vi "VNA_Easy_Loop.vi"(4 "Power (dbm)":dbl=-19.0, 5 "Transport":refnum<class "Transport.lvclass">, 6 "stop/span":dbl=600000000.0 format="%.2p", 7 "VNA Address":refnum<visa-resource-name>="GPIB0::15::INSTR", 8 "start/center":dbl=400000000.0 format="%.2p", 9 "sweep type (0 : linear)":u16(ring) items=["linear sweep", "logarithmic sweep", "frequency list", "CW time sweep", "power sweep"], 10 "sweep time (sec)":dbl=1.0 format="%.2f", 11 "num points":u16(ring)=8 items=["3", "11", "21 ('20) / 26 ('53)", "51", "101", "201", "401", "801", "1601"]) -> (2 "Polar plot":cluster{dbl[], sgl[]}[](graph))   [LabVIEW 2019]
uses:
  <userlib>/LevyLab/Transport/Transport/Transport.lvclass/Transport.ctl
  <userlib>/LevyLab/Transport/Control Experiment/Control Experiment.lvclass/Control Experiment.ctl
  <userlib>/LevyLab/Instrument Framework/Instrument Types/Cryostat/Instrument.Cryostat.lvclass
  <instrlib>/Agilent 87XX Series/Agilent 87XX Series.lvlib
  <userlib>/LevyLab/Transport/Control Experiment/Control Experiment.lvclass
  <userlib>/LevyLab/Transport/Transport/Transport.lvclass
panel:
  out "Data 2":cluster{dbl[], dbl[]}[](graph)
  out "B Field (T)":dbl=0.0002
  out "Temperature (K)":dbl=0.05877533421575553
  in  "Vg (V)":dbl
  in  "Ids (mA)":dbl=9.5
  in  "Vds (V)":dbl=1.3
  in  "Experiment Description":string="Vbg (1Gohm)=AO6 = P_pump = -20dBm to -5dBm, 0.1 dBm\n wait time 2s\nF_pump=2f0 = 900Mhz\n\nVbg(AO6) = 0V\nB=0T\nP_vna = -19.0 dBm (resonance at 488MHz with no pump)\n400MHz to 600MHz\nVd: 1.3V\nId: 9.5mA"
  in  "Experiment Folder":string="22-Vbgpump2f_Psweep_highPvna"
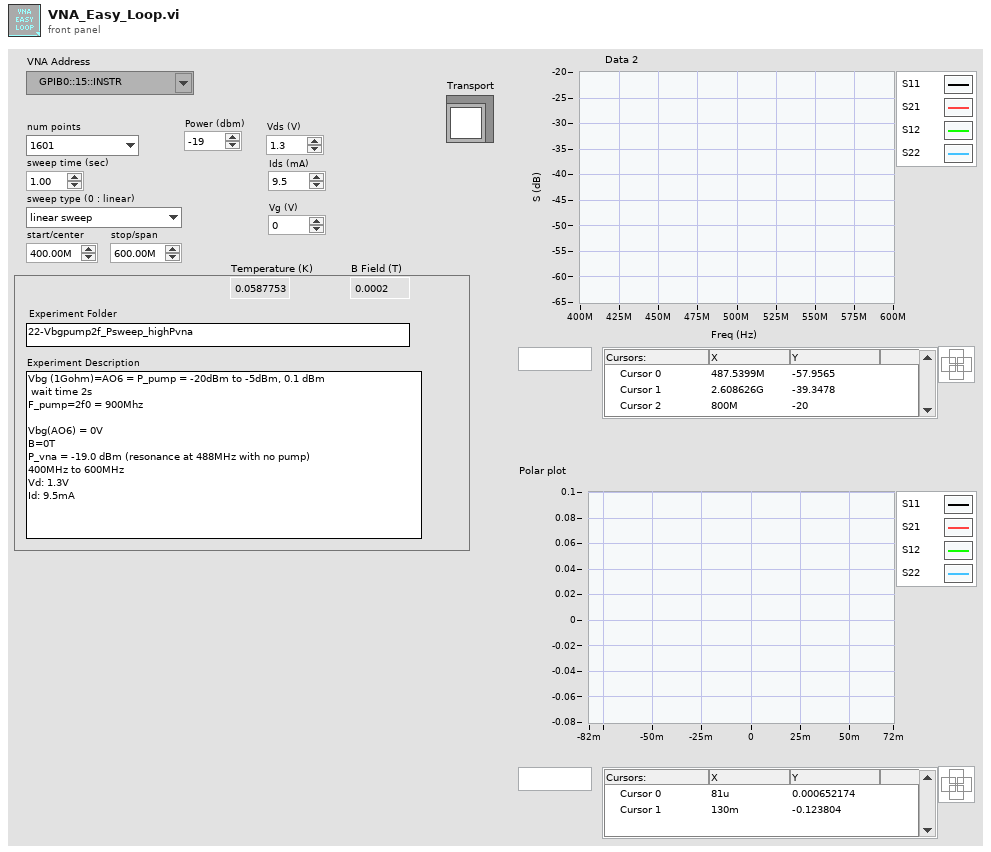
[diagram p1: front panel]
types:
  T1 = enum32{"Bad", "Idle", "Run top level", "Running"}
  T2 = typedef "Control Experiment.lvclass/Instruments--cluster.ctl" = cluster{"KH7008":refnum<class "Instrument.KH7008.lvclass">[], "Lockin":refnum<class "Instrument.Lockin.lvclass">, "Temperature":refnum<class "Instrument.Cryostat.lvclass">, "Magnet":refnum<class "Instrument.Cryostat.lvclass">, "Rotator":refnum<class "Instrument.Cryostat.lvclass">, "Level":refnum<class "Instrument.Cryostat.lvclass">, "Capacitance Bridge":refnum<class "Instrument.CBridge.lvclass">, "Delay Line":refnum<class "Instrument.DelayLine.lvclass">, "Strain Cell":refnum<class "Instrument.Strain.lvclass">, "VNA":refnum<class "Instrument.VNA.lvclass">, "Voltage Source":refnum<class "Instrument.VSource.lvclass">}
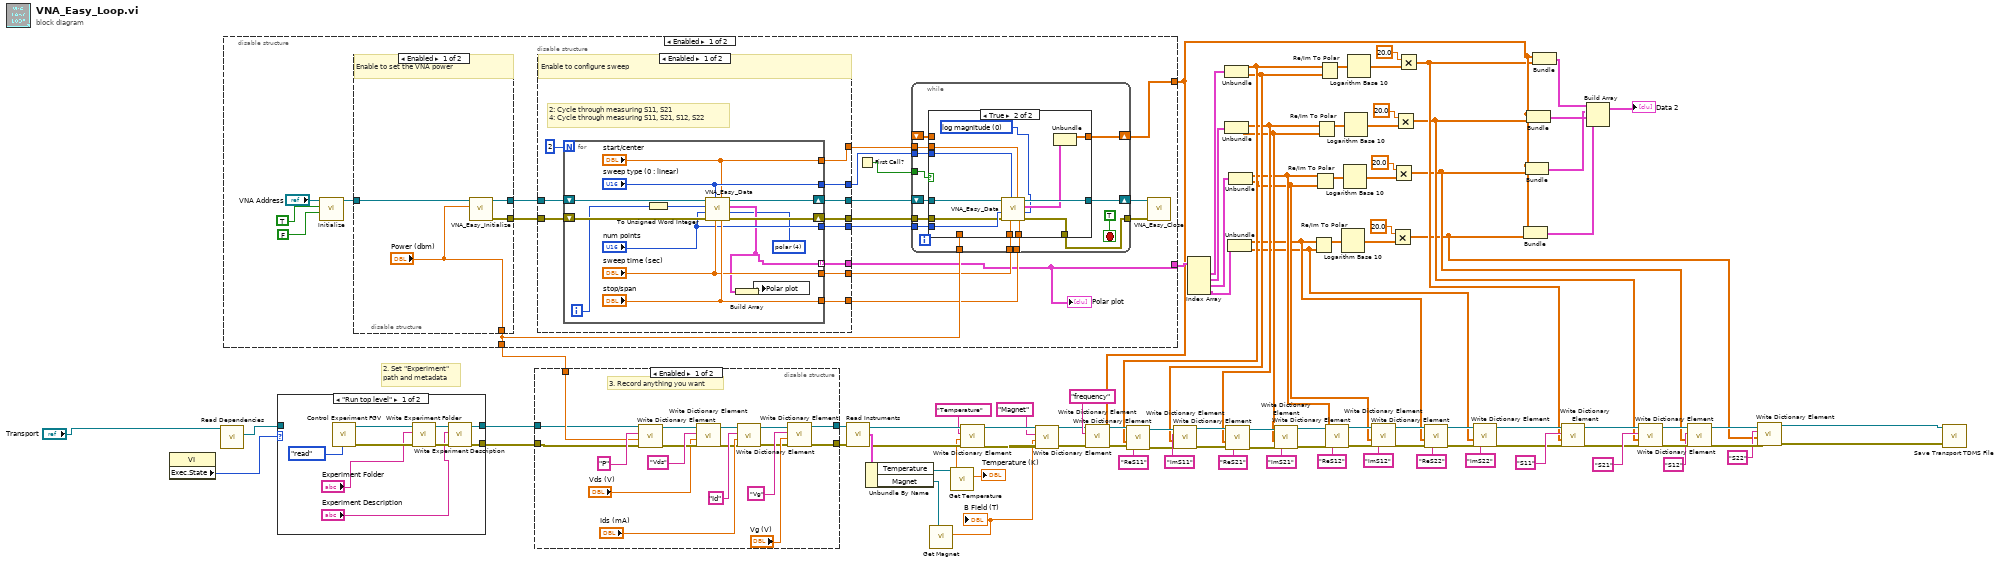
[diagram p0: block diagram]
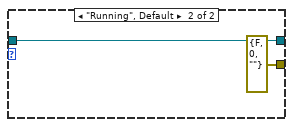
[diagram p2: hidden frame]
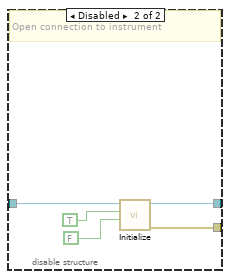
[diagram p5: hidden frame]
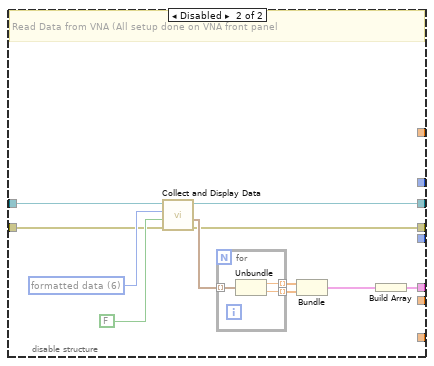
[diagram p6: hidden frame]
diagram:
  # "2. Set \"Experiment\"\npath and metadata"
  n1 = property class="VI"() -> ("Exec.State"=w62:T1)  [unwired: 2 in, 2 out]
  n2 = call <userlib>:"Read Dependencies.vi"("Transport"="Transport") -> ("C.E."=w58:refnum<class "Control Experiment.lvclass">)  [unwired: 8 in, 2 out]
  n3 = disable-structure shown="Enabled" {
    disable-tunnel: [w97 _] -> w57
    disable-tunnel: [w106 _] -> w88
    disable-tunnel: [w107 _] -> w15
    frame Enabled {
      n4 = call <instrlib>:"Initialize.vi"("reset"=FALSE, "ID query"=TRUE, "VISA resource name"="VNA Address") -> ("VISA resource name out"=w110:refnum<visa-resource-name>)  [unwired: 7 in, 1 out]
      n5 = disable-structure shown="Enabled" {
        disable-tunnel: w110 -> [w147 w150]
        disable-tunnel: [w146 w148] -> w114
        disable-tunnel: [w145 w149] -> w113
        disable-tunnel: ["Power (dbm)" _] -> w106
        frame Enabled {
          # "Enable to set the VNA power"
          n6 = call "VNA_Easy_Initialize.vi"("Power (dbm)"="Power (dbm)", "VISA Refnum in"=w147) -> ("error out"=w145:errorcluster, "VISA Refnum out"=w146:refnum<visa-resource-name>)  [unwired: 8 in]
        }
        frame Disabled {
          # "Open connection to instrument"
          n7 = call <instrlib>:"Initialize.vi"("reset"=FALSE, "ID query"=TRUE, "VISA resource name"=w150) -> ("error out"=w149:errorcluster, "VISA resource name out"=w148:refnum<visa-resource-name>)  [unwired: 7 in]
        }
      }
      n8 = disable-structure shown="Enabled" {
        disable-tunnel: w114 -> [w163 w182]
        disable-tunnel: w113 -> [w162 w183]
        disable-tunnel: [w161 w180] -> w105
        disable-tunnel: [w160 w181] -> w109
        disable-tunnel: [w159 w178] -> w97
        disable-tunnel: [w157 _] -> w103
        disable-tunnel: [w156 _] -> w102
        disable-tunnel: [w155 _] -> w101
        disable-tunnel: [w154 _] -> w100
        disable-tunnel: [w153 _] -> w99
        frame Enabled {
          # "2: Cycle through measuring S11, S21\n4: Cycle through measuring S11, S21, S12, S22"
          # "Enable to configure sweep"
          n9 = for {
            N: 2 -> [_]
            tunnel: [w165] -> w159 mode=indexing
            shift-right: [w174] -> w160
            shift-left: w163 -> [w177]
            shift-right: [w175] -> w161
            shift-left: w162 -> [w176]
            tunnel: ["sweep type (0 : linear)"] -> w157
            tunnel: ["stop/span"] -> w156
            tunnel: ["sweep time (sec)"] -> w155
            tunnel: ["start/center"] -> w154
            tunnel: ["num points"] -> w153
            i -> [w173]
            w164 = u16 4 items=["log magnitude", "phase", "delay", "Smith chart", "polar", "linear magnitude", "standing wave ratio", "real", "imaginary"] ("format (0 : log mag)")
            n10 = To Unsigned Word Integer(number=w173) -> (unsigned 16bit integer=w172:u16)
            n11 = call "VNA_Easy_Data.vi"("format (0 : log mag)"=w164, "stop/span"="stop/span", "start/center"="start/center", "sweep time (sec)"="sweep time (sec)", "sweep type (0 : linear)"="sweep type (0 : linear)", "error in (no error)"=w176, "num points"="num points", "measurement (0 : S11)"=w172, "VISA Refnum in"=w177) -> ("error out"=w175:errorcluster, "Data"=w165:cluster{dbl[], sgl[]}, "VISA Refnum out"=w174:refnum<visa-resource-name>)
            n12 = Build Array(w165) -> (w166:cluster{dbl[], sgl[]}[])
            n13 = local write "Polar plot"(w166) -> ()
          }
        }
        frame Disabled {
          w188 = u16 6 items=["raw data array 1", "raw data array 2", "raw data array 3", "raw data array 4", "error-corrected data", "error-corrected trace memory", "formatted data", "formatted memory", "formatted data / memory", "formatted data - memory"] ("data type (6 : formatted data)")
          # "Read Data from VNA (All setup done on VNA front panel"
          n14 = call <instrlib>:"Collect and Display Data.vi"("error in (no error)"=w183, "save to file"=FALSE, "data type (6 : formatted data)"=w188, "VISA resource name"=w182) -> ("error out"=w180:errorcluster, "data values"=w185:cluster{"real / stim":dbl, "imag / resp":sgl}[], "VISA resource name out"=w181:refnum<visa-resource-name>)  [unwired: 4 in, 1 out]
          n15 = for {
            tunnel: w185 -> [w191] mode=indexing
            tunnel: [w190] -> w186 mode=indexing
            tunnel: [w189] -> w187 mode=indexing
            n16 = Unbundle(w191) -> ("real / stim"=w190:dbl, "imag / resp"=w189:sgl)
          }
          n17 = Bundle(w186, w187) -> (w179:cluster{dbl[], sgl[]})  [unwired: 1 in]
          n18 = Build Array(w179) -> (w178:cluster{dbl[], sgl[]}[])
        }
      }
      "Polar plot" <- w97
      n19 = First Call?() -> (First Call?: T/F=w98:bool)
      n20 = while {
        shift-right: [w127] -> w108
        shift-left: w109 -> [w128]
        shift-right: [w125] -> w107
        shift-left: _ -> [w124]
        tunnel: w98 -> [w123]
        tunnel: w106 -> [w122]
        tunnel: w105 -> [w121]
        tunnel: [w120] -> w104
        tunnel: w103 -> [w119]
        tunnel: w102 -> [w118]
        tunnel: w101 -> [w117]
        tunnel: w100 -> [w116]
        tunnel: w99 -> [w115]
        stop <- TRUE stop-if-true
        n21 = case shown="True" w123 {
          tunnel: w128 -> [w130 w133]
          tunnel: [w130 w143] -> w127
          tunnel: [w131 w141] -> w125
          tunnel: w124 -> [w131 _]
          tunnel: w122 -> [_ _]
          tunnel: w121 -> [w129 w132]
          tunnel: [w129 w140] -> w120
          tunnel: w119 -> [_ w139]
          tunnel: w118 -> [_ w138]
          tunnel: w117 -> [_ w137]
          tunnel: w116 -> [_ w136]
          tunnel: w115 -> [_ w135]
          frame False {
          }
          frame True {
            w134 = u16 0 items=["log magnitude", "phase", "delay", "Smith chart", "polar", "linear magnitude", "standing wave ratio", "real", "imaginary"] ("format (0 : log mag)")
            n22 = call "VNA_Easy_Data.vi"("format (0 : log mag)"=w134, "stop/span"=w138, "start/center"=w136, "sweep time (sec)"=w137, "sweep type (0 : linear)"=w139, "error in (no error)"=w132, "num points"=w135, "VISA Refnum in"=w133) -> ("error out"=w140:errorcluster, "Data"=w142:cluster{dbl[], sgl[]}, "VISA Refnum out"=w143:refnum<visa-resource-name>)  [unwired: 1 in]
            n23 = Unbundle(w142) -> (w141:dbl[])  [unwired: 1 out]
          }
        }
      }
      n24 = call "VNA_Easy_Close.vi"("error in (no error)"=w104, "VISA Refnum in"=w108) -> ()  [unwired: 9 in, 1 out]
    }
    frame Disabled {
    }
  }
  n25 = case shown="\"Run top level\"" w62 {
    tunnel: [w196 errorcluster {"status"=FALSE, "code"=0, "source"=""} ("error out")] -> w60
    tunnel: [w195 w202] -> w61
    tunnel: w58 -> [_ w202]
    frame "Run top level" {
      n26 = call <userlib>:"Control Experiment FGV.vi"("Function"=enum16{"read", "write"}."read") -> ("error out"=w199:errorcluster, "Control Experiment.lvclass out"=w200:refnum<class "Control Experiment.lvclass">)  [unwired: 9 in]
      n27 = call <userlib>:"Write Experiment Folder.vi"("error in (no error)"=w199, "Experiment Folder"="Experiment Folder", "Control Experiment in"=w200) -> ("error out"=w197:errorcluster, "Control Experiment out"=w198:refnum<class "Control Experiment.lvclass">)  [unwired: 7 in]
      n28 = call <userlib>:"Write Experiment Description.vi"("error in (no error)"=w197, "Experiment Description"="Experiment Description", "Control Experiment in"=w198) -> ("error out"=w196:errorcluster, "Control Experiment out"=w195:refnum<class "Control Experiment.lvclass">)  [unwired: 7 in]
    }
    frame "Running", Default {
    }
  }
  n29 = disable-structure shown="Enabled" {
    disable-tunnel: w61 -> [w212 w222]
    disable-tunnel: w60 -> [w211 w221]
    disable-tunnel: [w217 w222] -> w87
    disable-tunnel: [w203 w221] -> w86
    disable-tunnel: w88 -> [w213 _]
    frame Enabled {
      # "3. Record anything you want"
      n30 = call <userlib>:"Write Dictionary Element.vi"("error in (no error)"=w211, "value"=w213, "key"="P", "Control Experiment in"=w212) -> ("error out"=w209:errorcluster, "Control Experiment out"=w210:refnum<class "Control Experiment.lvclass">)  [unwired: 6 in]
      n31 = call <userlib>:"Write Dictionary Element.vi"("error in (no error)"=w209, "value"="Vds (V)", "key"="Vds", "Control Experiment in"=w210) -> ("error out"=w206:errorcluster, "Control Experiment out"=w219:refnum<class "Control Experiment.lvclass">)  [unwired: 6 in]
      n32 = call <userlib>:"Write Dictionary Element.vi"("error in (no error)"=w206, "value"="Ids (mA)", "key"="Id", "Control Experiment in"=w219) -> ("error out"=w204:errorcluster, "Control Experiment out"=w218:refnum<class "Control Experiment.lvclass">)  [unwired: 6 in]
      n33 = call <userlib>:"Write Dictionary Element.vi"("error in (no error)"=w204, "value"="Vg (V)", "key"="Vg", "Control Experiment in"=w218) -> ("error out"=w203:errorcluster, "Control Experiment out"=w217:refnum<class "Control Experiment.lvclass">)  [unwired: 6 in]
    }
    frame Disabled {
    }
  }
  n34 = call <userlib>:"Read Instruments.vi"("error in (no error)"=w86, "Control Experiment in"=w87) -> ("error out"=w82:errorcluster, "Instruments"=w85:T2, "Control Experiment out"=w81:refnum<class "Control Experiment.lvclass">)  [unwired: 7 in]
  n35 = Unbundle By Name(w85) -> ("Temperature"=w83:refnum<class "Instrument.Cryostat.lvclass">, "Magnet"=w84:refnum<class "Instrument.Cryostat.lvclass">)
  n36 = call-dynamic "Get Magnet.vi"("Instrument.Cryostat in"=w84) -> ("B Field (T)"=w73:dbl)  [unwired: 6 in, 4 out]
  "B Field (T)" <- w73
  n37 = call-dynamic "Get Temperature.vi"("Instrument.Cryostat in"=w83) -> ("Temperature (K)"=w80:dbl)  [unwired: 6 in, 4 out]
  "Temperature (K)" <- w80
  n38 = call <userlib>:"Write Dictionary Element.vi"("error in (no error)"=w82, "value"=w80, "key"="Temperature", "Control Experiment in"=w81) -> ("error out"=w75:errorcluster, "Control Experiment out"=w78:refnum<class "Control Experiment.lvclass">)  [unwired: 6 in]
  n39 = call <userlib>:"Write Dictionary Element.vi"("error in (no error)"=w75, "value"=w73, "key"="Magnet", "Control Experiment in"=w78) -> ("error out"=w76:errorcluster, "Control Experiment out"=w77:refnum<class "Control Experiment.lvclass">)  [unwired: 6 in]
  n40 = call <userlib>:"Write Dictionary Element.vi"("error in (no error)"=w76, "value"=w15, "key"="frequency", "Control Experiment in"=w77) -> ("error out"=w47:errorcluster, "Control Experiment out"=w49:refnum<class "Control Experiment.lvclass">)  [unwired: 6 in]
  n41 = Index Array(array=w57) -> (element #1=w95:cluster{dbl[], sgl[]}, element #2=w89:cluster{dbl[], sgl[]}, element #3=w65:cluster{dbl[], sgl[]}, element #4=w63:cluster{dbl[], sgl[]})  [unwired: 4 in]
  n42 = Unbundle(w95) -> (w25:dbl[], w24:sgl[])
  n43 = call <userlib>:"Write Dictionary Element.vi"("error in (no error)"=w47, "value"=w25, "key"="ReS11", "Control Experiment in"=w49) -> ("error out"=w46:errorcluster, "Control Experiment out"=w48:refnum<class "Control Experiment.lvclass">)  [unwired: 6 in]
  n44 = call <userlib>:"Write Dictionary Element.vi"("error in (no error)"=w46, "value"=w24, "key"="ImS11", "Control Experiment in"=w48) -> ("error out"=w41:errorcluster, "Control Experiment out"=w43:refnum<class "Control Experiment.lvclass">)  [unwired: 6 in]
  n45 = Unbundle(w89) -> (w11:dbl[], w10:sgl[])
  n46 = call <userlib>:"Write Dictionary Element.vi"("error in (no error)"=w41, "value"=w11, "key"="ReS21", "Control Experiment in"=w43) -> ("error out"=w40:errorcluster, "Control Experiment out"=w42:refnum<class "Control Experiment.lvclass">)  [unwired: 6 in]
  n47 = Unbundle(w63) -> (w7:dbl[], w6:sgl[])
  n48 = Unbundle(w65) -> (w9:dbl[], w8:sgl[])
  n49 = call <userlib>:"Write Dictionary Element.vi"("error in (no error)"=w40, "value"=w10, "key"="ImS21", "Control Experiment in"=w42) -> ("error out"=w28:errorcluster, "Control Experiment out"=w29:refnum<class "Control Experiment.lvclass">)  [unwired: 6 in]
  n50 = Re/Im To Polar(2:w6, 3:w7) -> (1:w17:dbl[])  [unwired: 1 out]
  n51 = Re/Im To Polar(2:w8, 3:w9) -> (1:w20:dbl[])  [unwired: 1 out]
  n52 = Re/Im To Polar(2:w10, 3:w11) -> (1:w1:dbl[])  [unwired: 1 out]
  n53 = Re/Im To Polar(2:w24, 3:w25) -> (1:w53:dbl[])  [unwired: 1 out]
  n54 = call <userlib>:"Write Dictionary Element.vi"("error in (no error)"=w28, "value"=w9, "key"="ReS12", "Control Experiment in"=w29) -> ("error out"=w36:errorcluster, "Control Experiment out"=w37:refnum<class "Control Experiment.lvclass">)  [unwired: 6 in]
  n55 = Logarithm Base 10(1:w17) -> (0:w16:dbl[])
  n56 = Logarithm Base 10(1:w20) -> (0:w19:dbl[])
  n57 = Logarithm Base 10(1:w1) -> (0:w22:dbl[])
  n58 = Logarithm Base 10(1:w53) -> (0:w52:dbl[])
  n59 = call <userlib>:"Write Dictionary Element.vi"("error in (no error)"=w36, "value"=w8, "key"="ImS12", "Control Experiment in"=w37) -> ("error out"=w31:errorcluster, "Control Experiment out"=w33:refnum<class "Control Experiment.lvclass">)  [unwired: 6 in]
  n60 = Multiply(x=20.0, y=w16) -> (x*y=w2:dbl[])
  n61 = Multiply(x=20.0, y=w19) -> (x*y=w3:dbl[])
  n62 = Multiply(x=20.0, y=w22) -> (x*y=w4:dbl[])
  n63 = Multiply(x=20.0, y=w52) -> (x*y=w5:dbl[])
  n64 = call <userlib>:"Write Dictionary Element.vi"("error in (no error)"=w31, "value"=w7, "key"="ReS22", "Control Experiment in"=w33) -> ("error out"=w30:errorcluster, "Control Experiment out"=w32:refnum<class "Control Experiment.lvclass">)  [unwired: 6 in]
  n65 = call <userlib>:"Write Dictionary Element.vi"("error in (no error)"=w30, "value"=w6, "key"="ImS22", "Control Experiment in"=w32) -> ("error out"=w26:errorcluster, "Control Experiment out"=w27:refnum<class "Control Experiment.lvclass">)  [unwired: 6 in]
  n66 = Bundle(w15, w2) -> (w12:cluster{dbl[], dbl[]})  [unwired: 1 in]
  n67 = Bundle(w15, w3) -> (w13:cluster{dbl[], dbl[]})  [unwired: 1 in]
  n68 = Bundle(w15, w4) -> (w14:cluster{dbl[], dbl[]})  [unwired: 1 in]
  n69 = Bundle(w15, w5) -> (w56:cluster{dbl[], dbl[]})  [unwired: 1 in]
  n70 = call <userlib>:"Write Dictionary Element.vi"("error in (no error)"=w26, "value"=w5, "key"="S11", "Control Experiment in"=w27) -> ("error out"=w91:errorcluster, "Control Experiment out"=w90:refnum<class "Control Experiment.lvclass">)  [unwired: 6 in]
  n71 = Build Array(w56, w14, w13, w12) -> (→"Data 2":cluster{dbl[], dbl[]}[])
  n72 = call <userlib>:"Write Dictionary Element.vi"("error in (no error)"=w91, "value"=w4, "key"="S21", "Control Experiment in"=w90) -> ("error out"=w69:errorcluster, "Control Experiment out"=w72:refnum<class "Control Experiment.lvclass">)  [unwired: 6 in]
  n73 = call <userlib>:"Write Dictionary Element.vi"("error in (no error)"=w69, "value"=w3, "key"="S12", "Control Experiment in"=w72) -> ("error out"=w68:errorcluster, "Control Experiment out"=w71:refnum<class "Control Experiment.lvclass">)  [unwired: 6 in]
  n74 = call <userlib>:"Write Dictionary Element.vi"("error in (no error)"=w68, "value"=w2, "key"="S22", "Control Experiment in"=w71) -> ("error out"=w64:errorcluster, "Control Experiment out"=w70:refnum<class "Control Experiment.lvclass">)  [unwired: 6 in]
  n75 = call <userlib>:"Save Transport TDMS File.vi"("error in (no error)"=w64, "Control Experiment in"=w70) -> ()  [unwired: 8 in, 2 out]
